vi "Write Serial.vi"(8 "error in (no error)":errorcluster, 10 "Serial":string, 11 "ThAr in":refnum<class "ThAr.lvclass">) -> (0 "error out":errorcluster, 3 "ThAr out":refnum<class "ThAr.lvclass">)   [LabVIEW 2016, in "ThAr.lvclass"]
uses:
  ThAr.lvclass
  ThAr.lvclass/ThAr.ctl
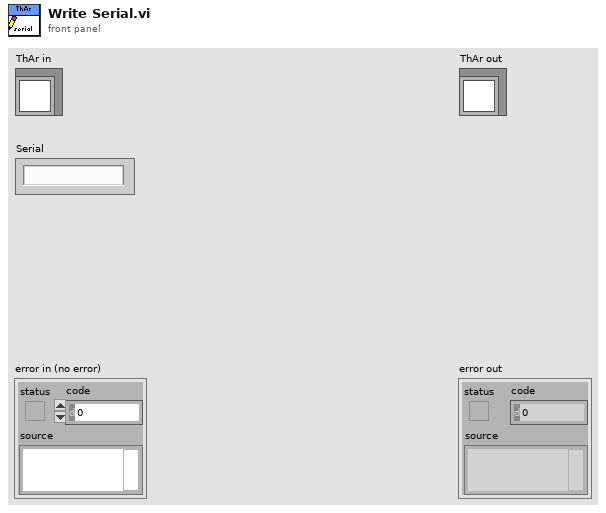
[diagram p1: front panel]
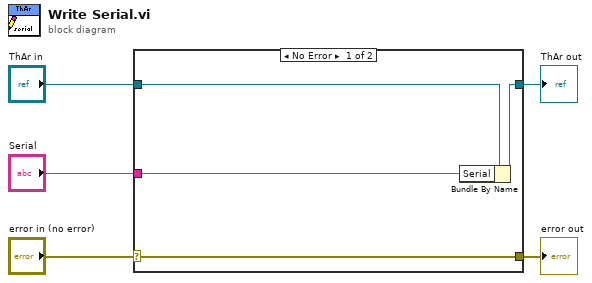
[diagram p0: block diagram]
diagram:
  n1 = case shown="No Error" "error in (no error)" {
    selector: "error in (no error)" -> [w9 w10]
    tunnel: [w9 w10] -> w4
    tunnel: [w7 w11] -> w2
    tunnel: "ThAr in" -> [w8 w11]
    tunnel: "Serial" -> [w6 _]
    frame No Error {
      n2 = Bundle By Name(cluster=w8, "Serial"=w6) -> (w7:refnum<class "ThAr.lvclass">)
    }
    frame Error {
    }
  }
  "error out" <- w4
  "ThAr out" <- w2
